vi "_059.vi"() -> ()   [LabVIEW 2024]
panel:
  in  "text":string
  out "error out":errorcluster
  out "appended path":path
  out "Application Directory":path
  # "To get proper Data (for each run ) :"
  # "( with proper date & time )"
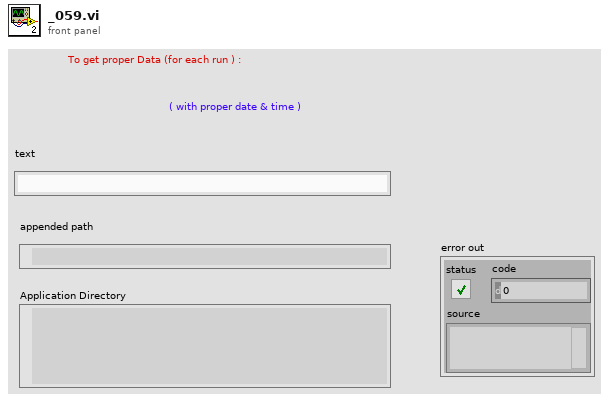
[diagram p1: front panel]
types:
  T1 = enum16{"open", "replace", "create", "open or create", "replace or create", "replace or create with confirmation"}
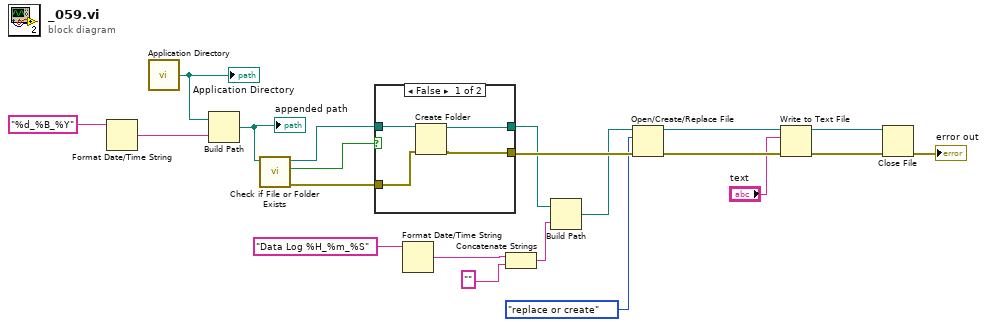
[diagram p0: block diagram]
diagram:
  n1 = Format Date/Time String(time format string (%c)="%d_%B_%Y") -> (date/time string=w20:string)  [unwired: 2 in]
  n2 = call <vilib>:"Application Directory.vi"() -> ("Application Directory"=w21:path)
  "Application Directory" <- w21
  n3 = Build Path(base path=w21, name or relative path=w20) -> (appended path=w17:path)
  "appended path" <- w17
  n4 = call <vilib>:"Check if File or Folder Exists.vi"("path"=w17) -> ("error out"=w15:errorcluster, "file or folder exists?"=w18:bool, "dup path"=w16:path)  [unwired: 8 in]
  n5 = case shown="False" w18 {
    tunnel: w16 -> [w25 w27]
    tunnel: [w24 w27] -> w6
    tunnel: [w23 w26] -> w12
    tunnel: w15 -> [w22 w26]
    frame False {
      n6 = Create Folder(path (use dialog)=w25, error in=w22) -> (created path=w24:path, error out=w23:errorcluster)  [unwired: 1 in, 1 out]
    }
    frame True {
    }
  }
  n7 = Format Date/Time String(time format string (%c)="Data Log %H_%m_%S") -> (date/time string=w5:string)  [unwired: 2 in]
  n8 = Concatenate Strings "Concatenate Strings"(w5, "" ("string")) -> (w3:string)
  n9 = Build Path(base path=w6, name or relative path=w3) -> (appended path=w2:path)
  n10 = Open/Create/Replace File(file path (use dialog)=w2, error in=w12, operation (0:open)=T1."replace or create") -> (refnum out=w11:refnum<file>, error out=w14:errorcluster)  [unwired: 3 in, 1 out]
  n11 = Write to Text File(file (use dialog)=w11, text="text", error in=w14) -> (refnum out=w10:refnum<file>, error out=w13:errorcluster)  [unwired: 1 in, 1 out]
  n12 = Close File(refnum=w10, error in=w13) -> (error out=→"error out":errorcluster)  [unwired: 1 out]
